vi "read_tt20_user_events.vi"(8 "error in (no error)":errorcluster, 11 "tt20panel in":refnum<class "tt20panel.lvclass">) -> (0 "error out":errorcluster, 2 "tt20_events":T1, 3 "tt20panel out":refnum<class "tt20panel.lvclass">)   [LabVIEW 2015, in "tt20panel.lvclass"]
uses:
  tt20panel.lvclass
  tt20_event_tdef.ctl
  tt20_class/tt20_hardware_info_tdef.ctl
  tt20_acq_mode_tdef.ctl
  tt20panel.lvclass/tt20panel.ctl
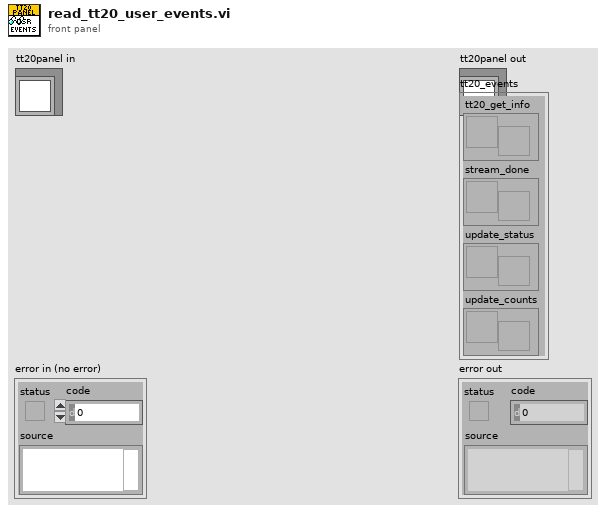
[diagram p1: front panel]
types:
  T1 = typedef "tt20_event_tdef.ctl" = cluster{"tt20_get_info":refnum<user-event>, "stream_done":refnum<user-event>, "update_status":refnum<user-event>, "update_counts":refnum<user-event>}
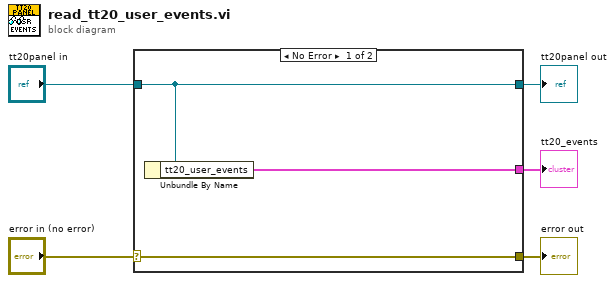
[diagram p0: block diagram]
diagram:
  n1 = case shown="No Error" "error in (no error)" {
    selector: "error in (no error)" -> [w8 w9]
    tunnel: [w8 w9] -> w4
    tunnel: [w7 w10] -> w2
    tunnel: "tt20panel in" -> [w7 w10]
    tunnel: [w6 _] -> w1
    frame No Error {
      n2 = Unbundle By Name(w7) -> ("tt20_user_events"=w6:T1)
    }
    frame Error {
    }
  }
  "error out" <- w4
  "tt20panel out" <- w2
  "tt20_events" <- w1
